vi "Charact One Point.vi"(0 "Scalar Path in":refnum<class "Scalar Path.lvclass">, 5 "Cal Point in":T1, 11 "error in (no error)":errorcluster) -> (4 "Scalar Path out":refnum<class "Scalar Path.lvclass">, 15 "error out":errorcluster)   [LabVIEW 2023, in "RFFixtureCharact.Public.lvlib" / "Scalar Path.lvclass"]
uses:
  Scalar Path.lvclass
  Type Definitions/Cal Point.ctl
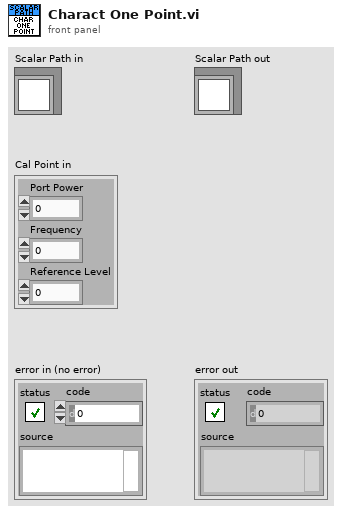
[diagram p1: front panel]
types:
  T1 = typedef "RFFixtureCharact.Public.lvlib/Scalar Path.lvclass/Cal Point.ctl" = cluster{"Port Power":dbl, "Frequency":dbl, "Reference Level":dbl}
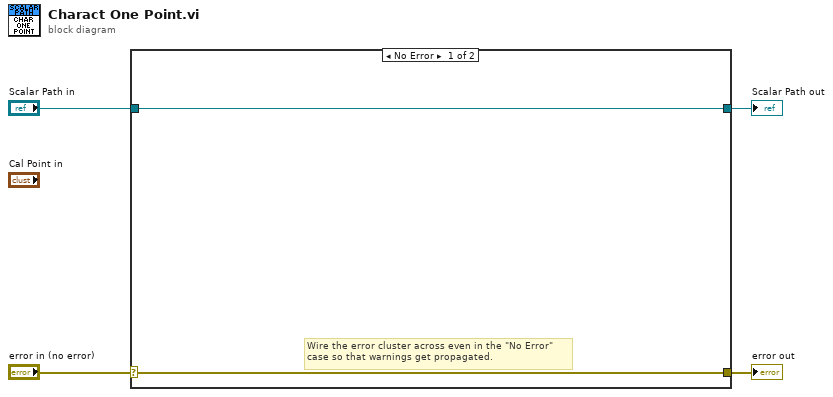
[diagram p0: block diagram]
diagram:
  n1 = case shown="No Error" "error in (no error)" {
    selector: "error in (no error)" -> [w5 w8]
    tunnel: [w5 w8] -> w3
    tunnel: [w6 w7] -> w1
    tunnel: "Scalar Path in" -> [w6 w7]
    frame No Error {
      # "Wire the error cluster across even in the \"No Error\"\ncase so that warnings get propagated."
    }
    frame Error {
    }
  }
  "error out" <- w3
  "Scalar Path out" <- w1
